vi "SR430_pause.vi"(0 "address":T1, 5 "error in (no error)":errorcluster) -> (14 "address out":T1, 19 "error out":errorcluster)   [LabVIEW 2015, in "SR430Driver.lvlib"]
doc: "Pauses (stops) a scan in progress. \n\nCopyright (C)\nGesellschaft für Schwerionenforschung, GSI\nPlanckstr. 1\n64291 Darmstadt\nGermany\n\nContact: D.Beck@gsi.de \n\nThis program is free software; you can redistribute it and/or modify it under the terms of the \nGNU General Public License as published by the Free Software Foundation; either version 2 of the license, or (at your option) any later version.\n\nThis program is distributed in the hope that it will be useful, but WITHOUT ANY WARRANTY; without even the implied warranty of MERCHANTABILITY or FITNESS FOR A PARTICULAR PURPOSE. See the GNU General License for more details (http://www.gnu.org).\n\nGesellschaft für Schwerionenforschung, GSI\nPlanckstr. 1, 64291 Darmstadt, Germany\nFor all questions and ideas contact: M.Richter@gsi.de, K.Poppensieker, H.Brand@gsi.de or D.Beck@gsi.de.\nLast update: 11-APR-2002"
uses:
  SR430Driver.lvlib
  SR430_VISA Control.ctl
panel:
  # "SR430 Pause"
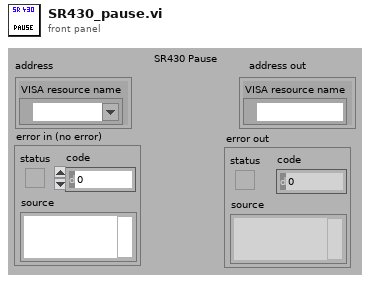
[diagram p1: front panel]
types:
  T1 = typedef "SR430Driver.lvlib/SR430_VISA Control.ctl" = cluster{"VISA resource name":refnum<visa-resource-name>}
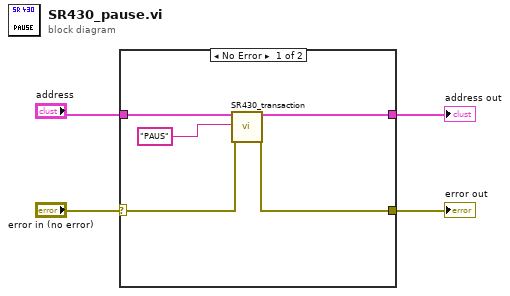
[diagram p0: block diagram]
diagram:
  n1 = case shown="No Error" "error in (no error)" {
    selector: "error in (no error)" -> [w7 w10]
    tunnel: "address" -> [w9 w11]
    tunnel: [w8 w11] -> w1
    tunnel: [w6 w10] -> w3
    frame No Error {
      n2 = call "SR430_transaction.vi"("SR430 VISA Cluster"=w9, "SR430 Command String"="PAUS", "error in (no error)"=w7) -> ("dup SR430 VISA Cluster"=w8:T1, "error out"=w6:errorcluster)  [unwired: 13 in, 2 out]
    }
    frame Error {
    }
  }
  "error out" <- w3
  "address out" <- w1
